vi "Overlay Cross.vi"() -> (3 "Image Out":T1)   [LabVIEW 2015]
uses:
  <vilib>/vision/Image Controls.llb/IMAQ Image.ctl
  Host Globals.vi
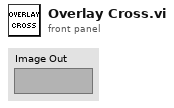
[diagram p1: front panel]
types:
  T1 = typedef "IMAQ Image.ctl" = refnum<image>
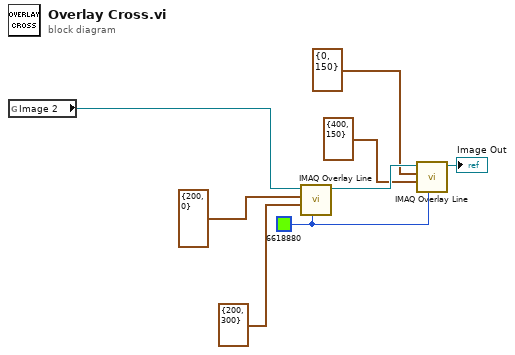
[diagram p0: block diagram]
diagram:
  w1 = u32 6618880 ("Color")
  n1 = global read "Host Globals.vi" "Image 2"() -> (w8:T1)
  n2 = call "IMAQ Overlay Line"("Color"=w1, "End Point"=cluster{"X":i32, "Y":i32} {"X"=200, "Y"=300}, "Start Point"=cluster{"X":i32, "Y":i32} {"X"=200, "Y"=0}, "Image"=w8) -> ("Image Out"=w7:T1)  [unwired: 6 in, 1 out]
  n3 = call "IMAQ Overlay Line"("Color"=w1, "End Point"=cluster{"X":i32, "Y":i32} {"X"=400, "Y"=150}, "Start Point"=cluster{"X":i32, "Y":i32} {"X"=0, "Y"=150}, "Image"=w7) -> ("Image Out"=→"Image Out":T1)  [unwired: 6 in, 1 out]
